vi "Page.vi"(8 "error in":errorcluster, 11 "Gen Refnum":refnum<vi>) -> (0 "error out":errorcluster, 3 "Page out":refnum<class "Page.lvclass">)   [LabVIEW 2014, in "Page.lvclass"]
uses:
  Page.lvclass
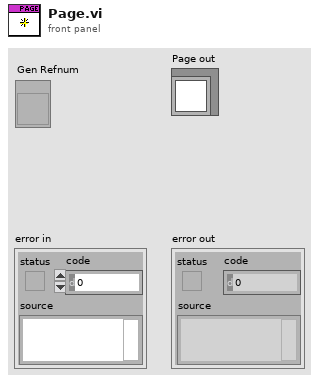
[diagram p1: front panel]
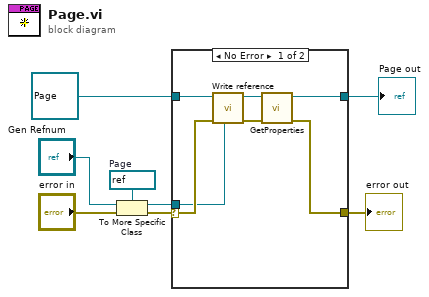
[diagram p0: block diagram]
diagram:
  w8 = refnum<vi> refnum  # Page
  n1 = To More Specific Class(target class=w8, reference="Gen Refnum", error in="error in") -> (specific class reference=w4:refnum<vi>, error out=w5:errorcluster)
  n2 = case shown="No Error" w5 {
    selector: w5 -> [w14 w17]
    tunnel: w4 -> [w13 _]
    tunnel: refnum<class "Page.lvclass"> refnum ("Page in") -> [w15 w16]
    tunnel: [w11 w16] -> w2
    tunnel: [w9 w17] -> w1
    frame No Error {
      n3 = call-dynamic "Write reference.vi"("reference"=w13, "error in"=w14, "GObject in"=w15) -> ("error out"=w10:errorcluster, "GObject out"=w12:refnum<class "Page.lvclass">)  [unwired: 5 in]
      n4 = call-dynamic "GetProperties.vi"("error in"=w10, "Page in"=w12) -> ("error out"=w9:errorcluster, "Page out"=w11:refnum<class "Page.lvclass">)  [unwired: 8 in]
    }
    frame Error {
    }
  }
  "error out" <- w1
  "Page out" <- w2
